vi "GCode Parser - SoftMotion Example.vi"() -> ()   [LabVIEW 2017]
uses:
  Typedefs/Motion Parameters.ctl
  <vilib>/Motion/Express/_s/nimc.fb.straightLineMove.blendMode.ctl
  GCode Parser/GCode Command Cluster.ctl
  <vilib>/Math Plots/3D Math Plots/3D Scatter/3D Scatter XCtrl/3D Scatter.xctl
  <vilib>/Motion/Express/_s/nimc.ex.clearFaults.clearFaults.axis.vi
  <vilib>/Motion/Express/_s/nimc.ex.power.power.axis.vi
  <vilib>/Motion/Express/_s/nimc.ex.resetPosition.resetPosition.axis.vi
  <vilib>/Motion/Express/_s/nimc.ex.straightLineMove.startStraightLineMove.coordinate.modeAbsolute.blendEnable.1.vi
  <vilib>/Motion/Express/_s/nimc.ex.arcMove.startArcMove.coordinate.modeCircular.blendEnable.1.vi
  <vilib>/Motion/Express/_s/nimc.ex.stopMove.stop.coordinate.modeDecelerate.vi
  <vilib>/Motion/Express/_s/nimc.ex.read.readTrajectoryData.coordinate.vi
  <vilib>/Motion/Express/_s/nimc.ex.read.readExecutionData.axis.vi
  <vilib>/Math Plots/3D Math Plots/3D Scatter/3D Scatter Datatype/Public/Plot Helper (Vector).vi
  <vilib>/Motion/BlockNode/FB.NIMotion.xnode
  <vilib>/Motion/Express/_s/nimc.fb.arcMove.blendMode.ctl
  <vilib>/Math Plots/3D Math Plots/3D Scatter/3D Scatter Datatype/3D Scatter Datatype.lvclass
panel:
  out "Array 2":string[](array[string])
  out "3D Scatter":refnum<class "3D Plot Datatype.lvclass">[](xcontrol)
  out "Array":dbl[](array[numeric])
  out "Current GCode Command":T1
  in  "Motion Parameters":T2={"timeout"=-1.0, "acceleration"=10000.0, "deceleration"=10000.0, "accel. jerk"=100000.0, "decel. jerk"=100000.0, "blend mode"=10551334, "blend delay"=-1.0, "smoothing"=0.5, "last blend"=FALSE} {"blend mode" items=["At Profile Complete"=10551335, "At Deceleration"=10551334, "After Delay"=10551336]}
  in  "G0 Velocity":dbl=20.0
  in  "Position Scale":dbl=1.0
  in  "Velocity Scale":dbl=1.0
  out "Global Stop":bool
  out "text":string
  in  "Quit":bool
  out "Iterations":i32
  out "Command Array":T1[](array[typedef])
  out "error out":errorcluster
  in  "start index":i32
  # "Be sure select \nafter delay"
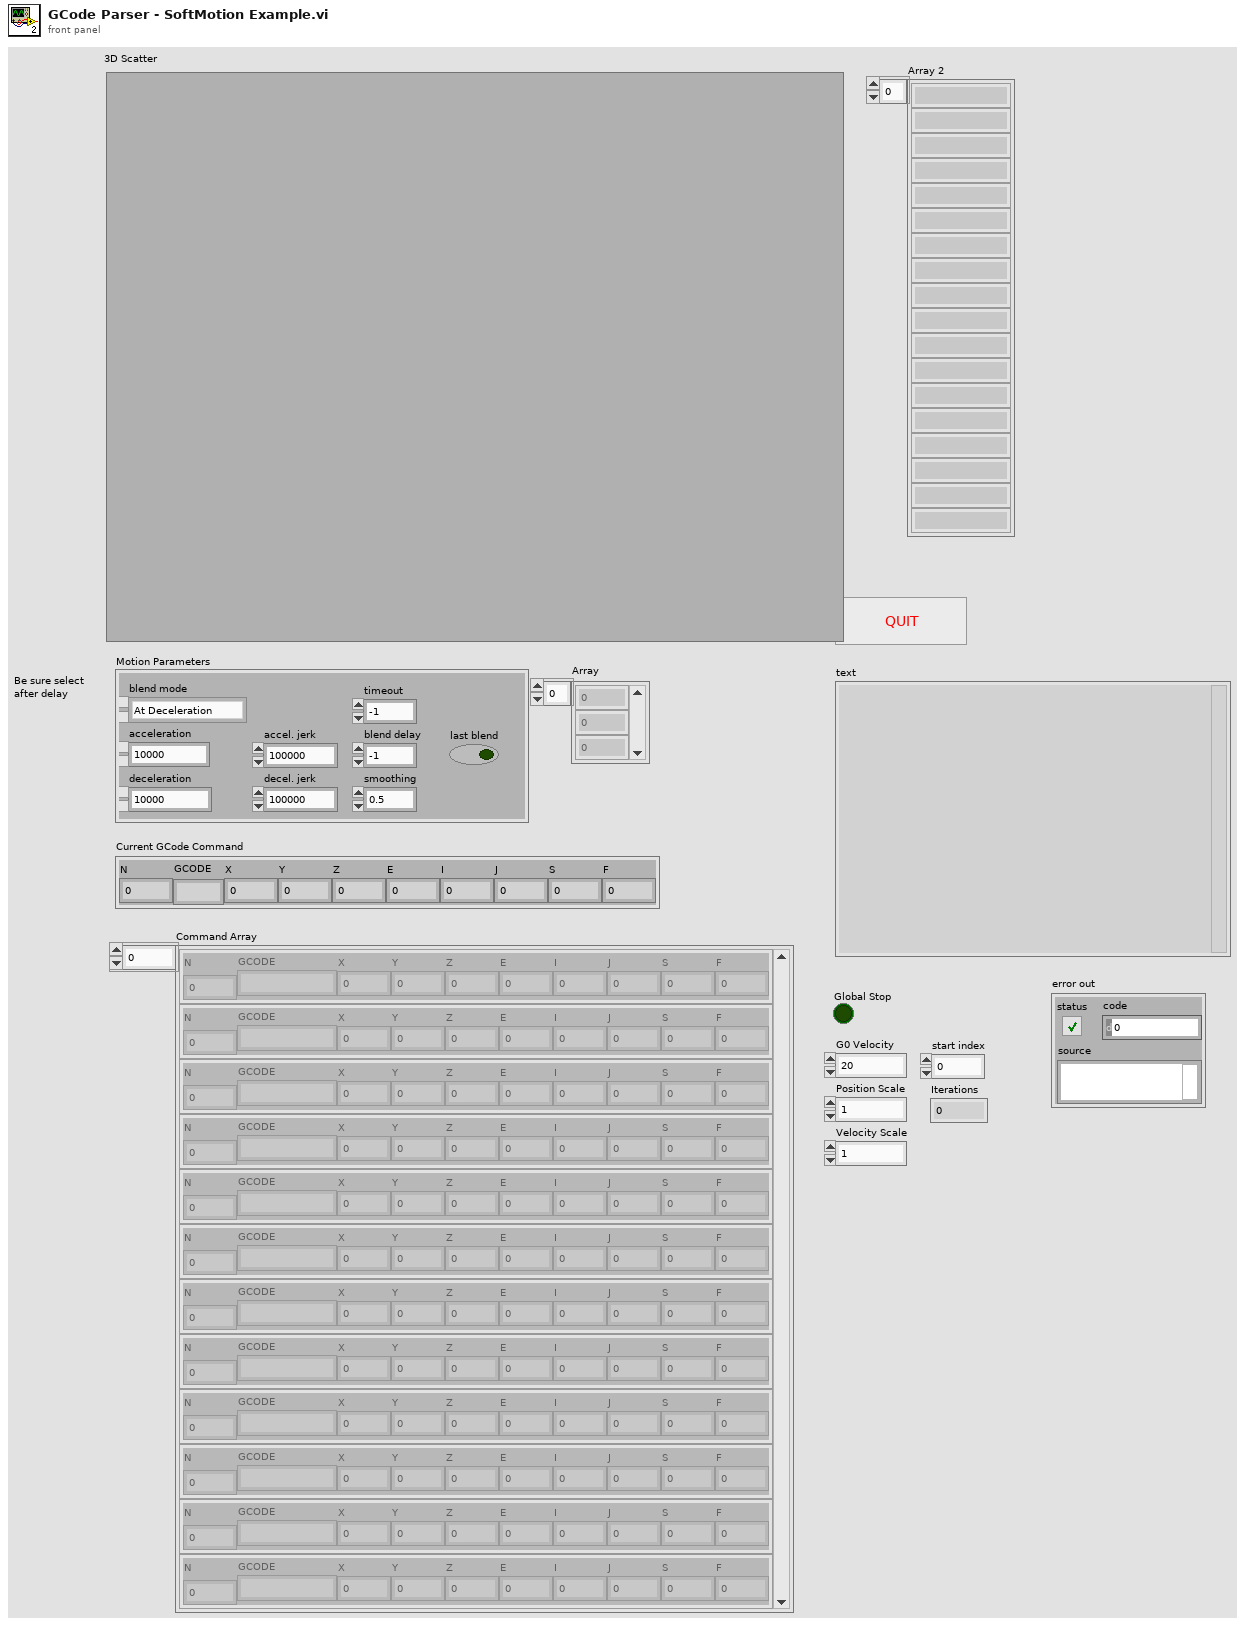
[diagram p1: front panel]
types:
  T1 = typedef "GCode Command Cluster.ctl" = cluster{"N":dbl, "GCODE":string, "X":dbl, "Y":dbl, "Z":dbl, "E":dbl, "I":dbl, "J":dbl, "S":dbl, "F":dbl}
  T2 = typedef "Motion Parameters.ctl" = cluster{"timeout":dbl, "acceleration":dbl, "deceleration":dbl, "accel. jerk":dbl, "decel. jerk":dbl, "blend mode":T3, "blend delay":dbl, "smoothing":dbl, "last blend":bool}
  T3 = typedef "nimc.fb.straightLineMove.blendMode.ctl" = i32
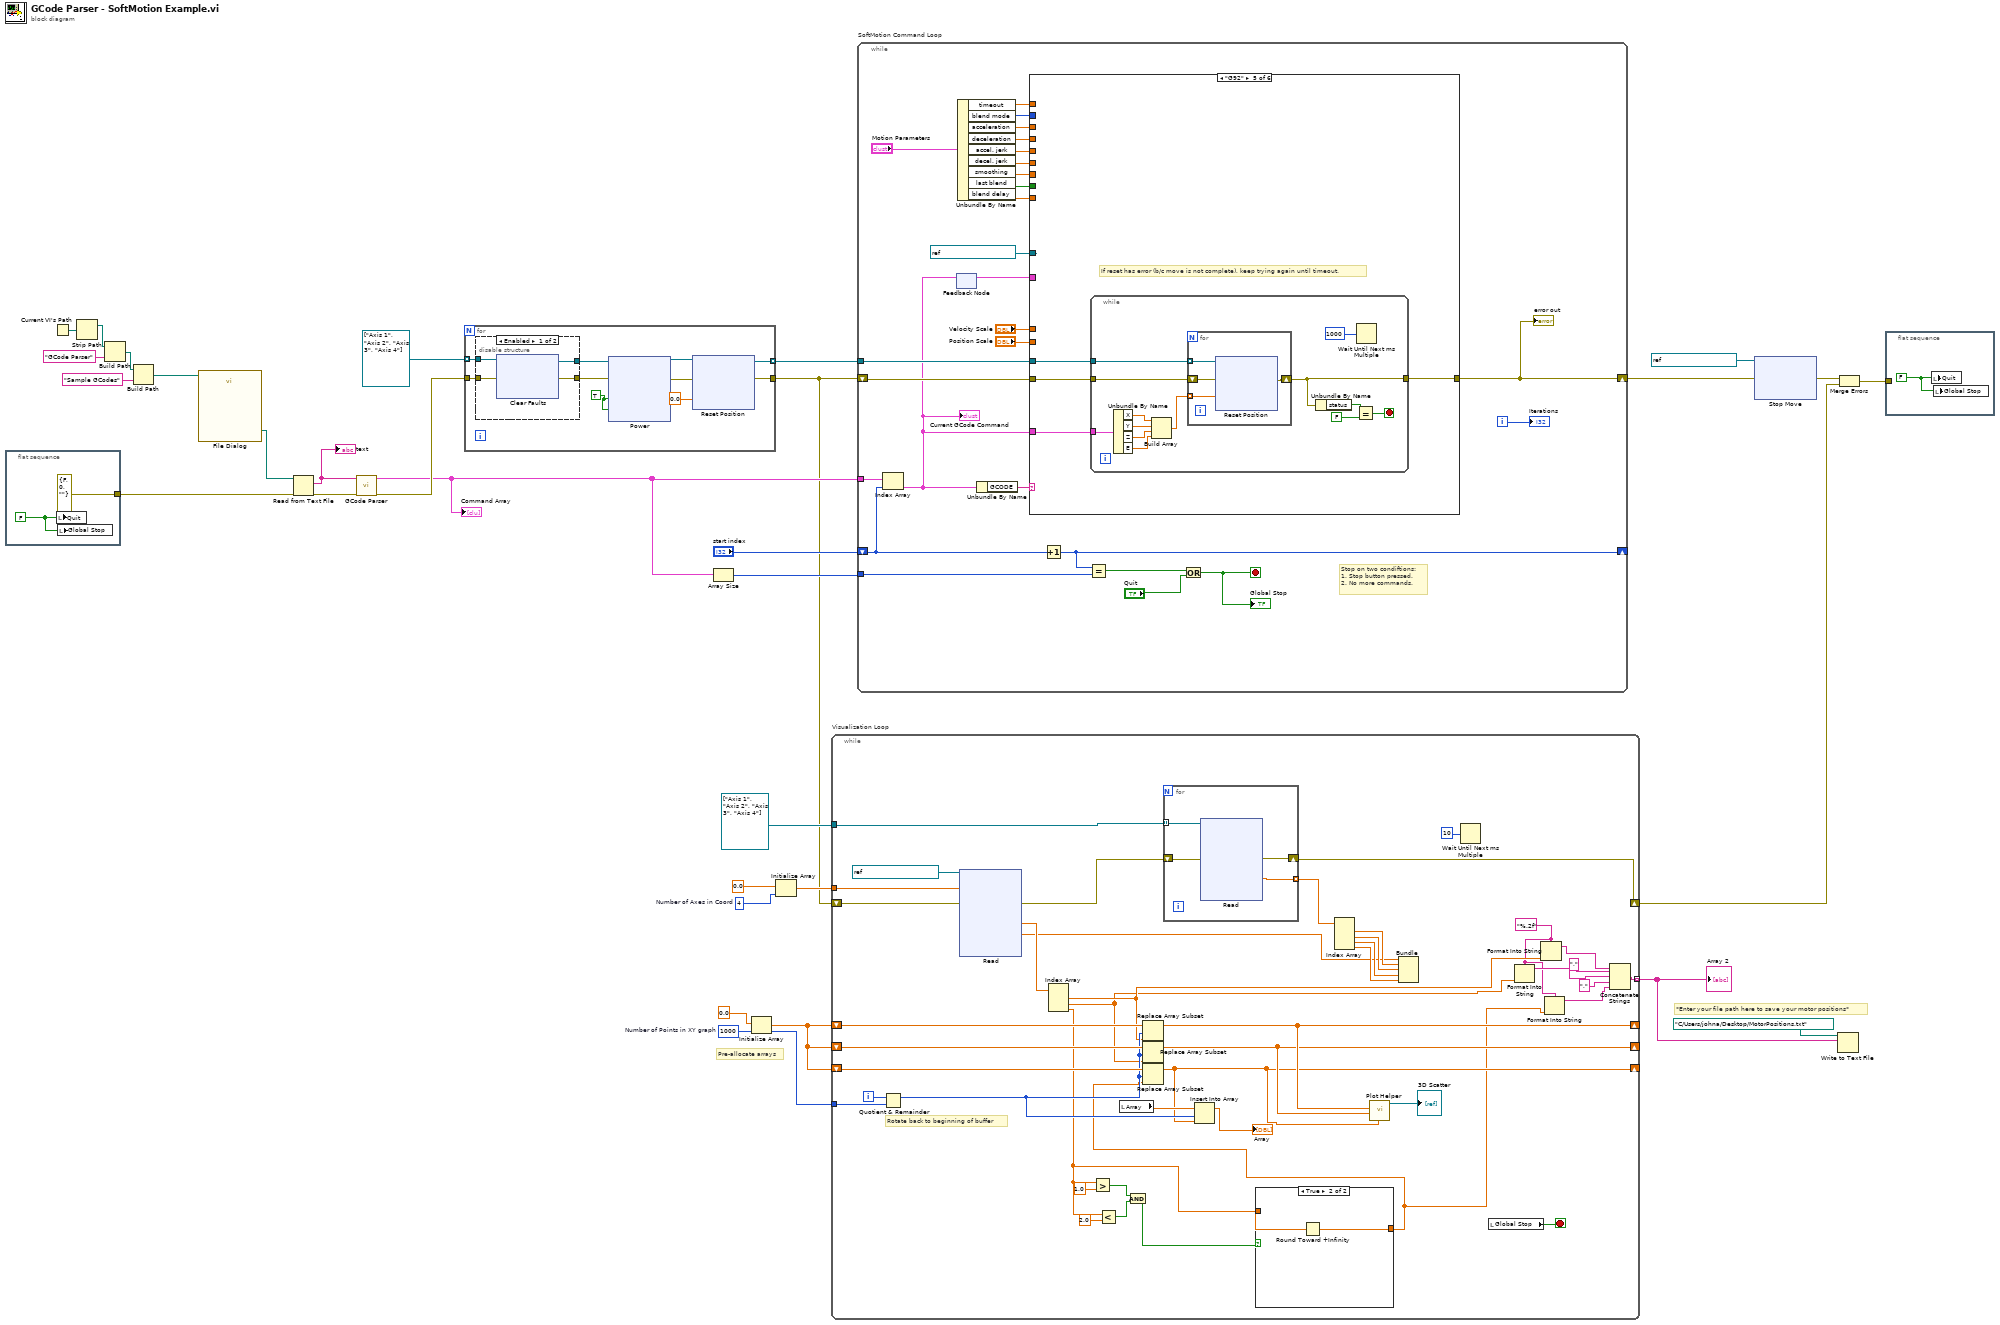
[diagram p0: block diagram]
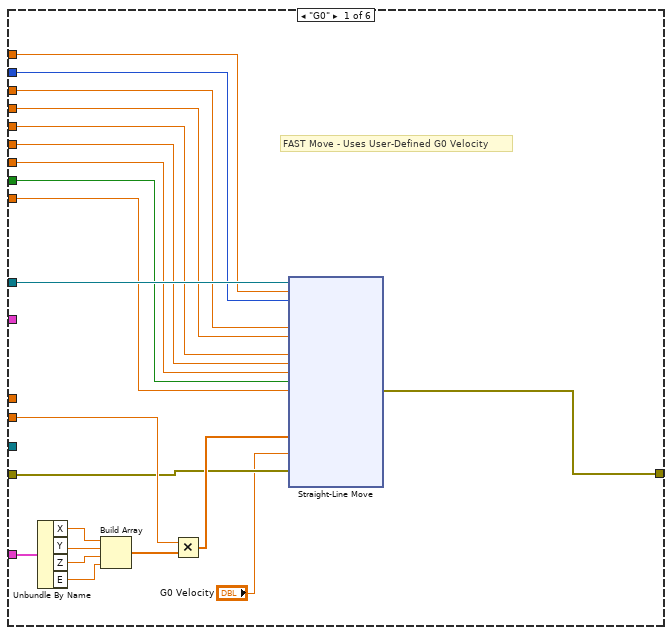
[diagram p2: hidden frame]
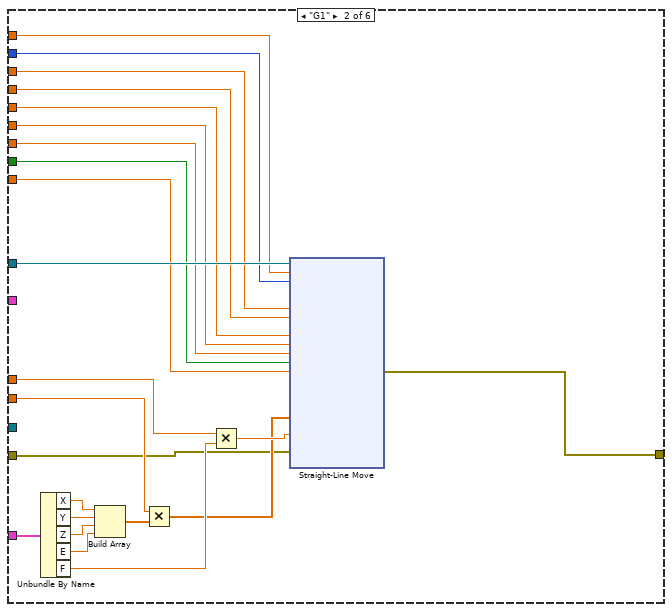
[diagram p3: hidden frame]
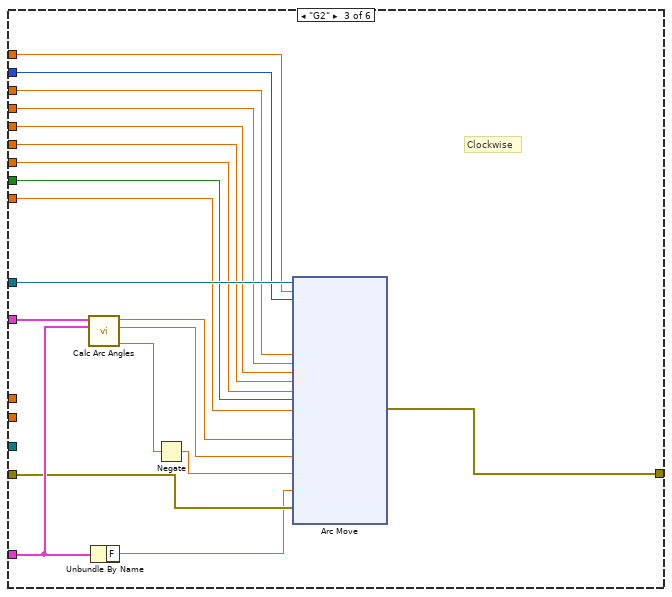
[diagram p4: hidden frame]
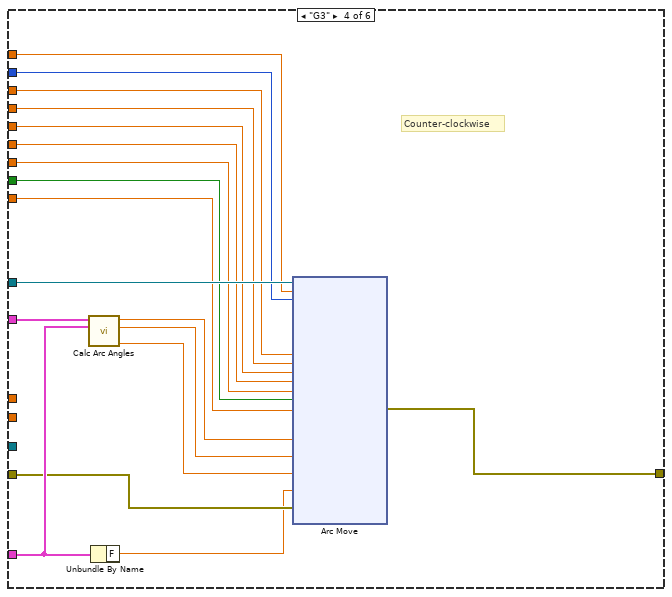
[diagram p5: hidden frame]
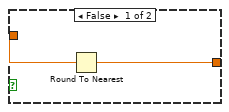
[diagram p7: hidden frame]
diagram:
  w27 = 1000  # Number of Points in XY graph
  w29 = 4  # Number of Axes in Coord
  # "*Enter your file path here to save your motor positions*"
  # "Pre-allocate arrays"
  n1 = flat-sequence {
    tunnel: [errorcluster {"status"=FALSE, "code"=0, "source"=""} ("error out")] -> w22
    frame #0 {
      w32 = FALSE ("Example Done")
      n2 = local write "Quit"(w32) -> ()
      n3 = local write "Global Stop"(w32) -> ()
    }
  }
  n4 = Current VI's Path() -> (path=w9:path)
  n5 = Strip Path(path=w9) -> (stripped path=w8:path)  [unwired: 1 out]
  n6 = Build Path(base path=w8, name or relative path="GCode Parser") -> (appended path=w4:path)
  n7 = Build Path(base path=w4, name or relative path="Sample GCodes") -> (appended path=w3:path)
  n8 = call "File Dialog"("start path"=w3) -> ("selected path"=w6:path)  [unwired: 11 in, 3 out]
  n9 = Read from Text File(file (use dialog)=w6, error in=w22) -> (text=w24:string, error out=w23:errorcluster)  [unwired: 2 in, 2 out]
  "text" <- w24
  n10 = call "GCode Parser.vi"("error in (no error)"=w23, "String in"=w24) -> ("error out"=w21:errorcluster, "Command Array"=w17:T1[])  [unwired: 8 in]
  "Command Array" <- w17
  n11 = for {
    tunnel: refnum<k21>[] ["Axis 1", "Axis 2", "Axis 3", "Axis 4"] -> [w43] mode=indexing
    tunnel: w21 -> [w42]
    tunnel: [w41] -> w14
    tunnel: [w34] -> w18 mode=indexing
    w36 = TRUE ("enable axis")
    n12 = disable-structure shown="Enabled" {
      disable-tunnel: w43 -> [w47 w53]
      disable-tunnel: w42 -> [w46 w52]
      disable-tunnel: [w45 w53] -> w39
      disable-tunnel: [w44 w52] -> w37
      frame Enabled {
        n13 = xnode ("Clear Faults")("resource"=w47, "error in"=w46) -> ("resource out"=w45:refnum<k21>, "error out"=w44:errorcluster)
      }
      frame Disabled {
      }
    }
    n14 = xnode ("Power")("enable axis"=w36, "enable drive"=w36, "resource"=w39, "error in"=w37) -> ("resource out"=w38:refnum<k21>, "error out"=w35:errorcluster)
    n15 = xnode ("Reset Position")("position"=0.0, "resource"=w38, "error in"=w35) -> ("resource out"=w34:refnum<k21>, "error out"=w41:errorcluster)
  }
  n16 = Array Size(array=w17) -> (size(s)=w16:i32)
  n17 = Initialize Array(0.0 ("element"), w27) -> (w26:dbl[])
  n18 = Initialize Array(0.0 ("element"), w29) -> (w25:dbl[])
  n19 = while "Visualization Loop" {
    shift-right: [w82] -> _
    shift-left: w26 -> [w110]
    shift-right: [w94] -> w13
    shift-left: w14 -> [w102]
    shift-right: [w81] -> _
    shift-left: w26 -> [w109]
    tunnel: w27 -> [w108]
    shift-right: [w80] -> _
    shift-left: w26 -> [w93]
    tunnel: w25 -> [w99]
    tunnel: refnum<k21>[] ["Axis 1", "Axis 2", "Axis 3", "Axis 4"] -> [w107]
    tunnel: [w76] -> w2 mode=indexing
    i -> [w91]
    stop <- w96 stop-if-true
    w69 = "%.2f" ("format string")
    # "Rotate back to beginning of buffer"
    n20 = Quotient & Remainder(x=w91, y=w108) -> (x-y*floor(x/y)=w89:i32)  [unwired: 1 out]
    n21 = xnode ("Read")("resource"=refnum<k21> "Coordinate Space 1" ("Motion Resource"), "commanded pos.[]"=w99, "error in"=w102) -> ("commanded pos.[] out"=w100:dbl[], "commanded vel."=w97:dbl, "error out"=w101:errorcluster)  [unwired: 3 out]
    n22 = Index Array(array=w100) -> (element #1=w75:dbl, element #2=w73:dbl, element #3=w79:dbl)  [unwired: 3 in]
    n23 = Greater?(x=w79, y=1.0) -> (0:w86:bool)
    n24 = Less?(x=w79, y=2.0) -> (x < y?=w85:bool)
    n25 = local read "Array"() -> (w90:dbl[])
    n26 = And(x=w86, y=w85) -> (x .and. y?=w84:bool)
    n27 = Replace Array Subset(array=w110, new element=w75, index=w89) -> (w82:dbl[])
    n28 = Replace Array Subset(array=w109, new element=w73, index=w89) -> (w81:dbl[])
    n29 = for {
      tunnel: w107 -> [w128] mode=indexing
      tunnel: [w127] -> w106 mode=indexing
      shift-right: [w125] -> w94
      shift-left: w101 -> [w126]
      n30 = xnode ("Read")("resource"=w128, "error in"=w126) -> ("velocity"=w127:dbl, "error out"=w125:errorcluster)  [unwired: 5 out]
    }
    n31 = case shown="True" w84 {
      tunnel: w79 -> [w113 w115]
      tunnel: [w112 w114] -> w71
      frame False {
        n32 = Round To Nearest(number=w113) -> (nearest integer value=w112:dbl)
      }
      frame True {
        n33 = Round Toward +Infinity(x=w115) -> (ceil(x): smallest int >= x=w114:dbl)
      }
    }
    n34 = Replace Array Subset(array=w93, new element=w71, index=w89) -> (w80:dbl[])
    n35 = Insert Into Array(array=w90, index=w89, new element=w80) -> (→"Array":dbl[])
    n36 = Index Array(array=w106) -> (element #1=w105:dbl, element #2=w104:dbl, element #3=w103:dbl, element #4=w98:dbl)  [unwired: 4 in]
    n37 = call-poly <vilib>:"Plot Helper.vi"("z vector"=w80, "y vector"=w81, "x vector"=w82) -> ("3D Plot lvclass Array out"=→"3D Scatter":refnum<class "3D Plot Datatype.lvclass">[])  [unwired: 3 in, 5 out]
    n38 = Bundle("commanded vel."=w97, "velocity"=w105, "velocity"=w104, "velocity"=w103, "velocity"=w98) -> ()  [unwired: 1 in, 1 out]
    n39 = Wait Until Next ms Multiple(millisecond multiple=u32 10) -> ()  [unwired: 1 out]
    n40 = local read "Global Stop"() -> (w96:bool)
    n41 = Format Into String(format string=w69, w73) -> (resulting string=w72:string)  [unwired: 2 in, 1 out]
    n42 = Format Into String(format string=w69, w75) -> (resulting string=w74:string)  [unwired: 2 in, 1 out]
    n43 = Format Into String(format string=w69, w71) -> (resulting string=w70:string)  [unwired: 2 in, 1 out]
    n44 = Concatenate Strings(w74, "," ("element"), w72, "," ("element"), w70) -> (w76:string)
  }
  "Array 2" <- w2
  n45 = while "SoftMotion Command Loop" {
    tunnel: w17 -> [w157]
    shift-right: [w154] -> _
    shift-left: "start index" -> [w156]
    shift-right: [w161] -> w11
    shift-left: w14 -> [w160]
    tunnel: w18 -> [w159]
    tunnel: w16 -> [w155]
    i -> [w158]
    stop <- w152 stop-if-true
    # "Stop on two condiftions:\n1. Stop button pressed.\n2. No more commands."
    n46 = Index Array(array=w157, index=w156) -> (element=w138:T1)
    "Current GCode Command" <- w138
    n47 = feedback-in #1(w138) -> ()
    n48 = feedback #1() -> (w139:T1)  [unwired: 1 in]
    n49 = Unbundle By Name("Motion Parameters") -> ("timeout"=w148:dbl, "blend mode"=w147:T3, "acceleration"=w146:dbl, "deceleration"=w145:dbl, "accel. jerk"=w144:dbl, "decel. jerk"=w143:dbl, "smoothing"=w141:dbl, "last blend"=w142:bool, "blend delay"=w140:dbl)
    n50 = Unbundle By Name(w138) -> ("GCODE"=w164:string)
    n51 = case shown="\"G92\"" w164 {
      tunnel: refnum<k21> "Coordinate Space 1" ("Motion Resource") -> [w177 w219 w267 w307 _ _]
      tunnel: [w185 w228 w257 w297 w330 w356] -> w161
      tunnel: "Velocity Scale" -> [_ w207 _ _ _ _]
      tunnel: w138 -> [w180 w223 w264 w304 w331 _]
      tunnel: "Position Scale" -> [w178 w220 _ _ _ _]
      tunnel: w160 -> [w175 w217 w258 w298 w332 w356]
      tunnel: w148 -> [w174 w216 w263 w303 _ _]
      tunnel: w147 -> [w173 w215 w249 w291 _ _]
      tunnel: w146 -> [w172 w214 w262 w302 _ _]
      tunnel: w145 -> [w171 w213 w261 w301 _ _]
      tunnel: w144 -> [w170 w212 w260 w300 _ _]
      tunnel: w143 -> [w169 w211 w259 w299 _ _]
      tunnel: w141 -> [w168 w210 w250 w292 _ _]
      tunnel: w142 -> [w167 w209 w251 w293 _ _]
      tunnel: w140 -> [w166 w208 w252 w294 _ _]
      tunnel: w159 -> [_ _ _ _ w333 _]
      tunnel: w139 -> [_ _ w266 w306 _ _]
      frame "G0" {
        # "FAST Move - Uses User-Defined G0 Velocity"
        n52 = Unbundle By Name(w180) -> ("X"=w184:dbl, "Y"=w183:dbl, "Z"=w182:dbl, "E"=w181:dbl)
        n53 = Build Array(w184, w183, w182, w181) -> (w179:dbl[])
        n54 = Multiply(x=w178, y=w179) -> (x*y=w176:dbl[])
        n55 = xnode ("Straight-Line Move")("position[]"=w176, "velocity"="G0 Velocity", "error in"=w175, "resource"=w177, "timeout"=w174, "blend mode"=w173, "acceleration"=w172, "deceleration"=w171, "accel. jerk"=w170, "decel. jerk"=w169, "smoothing"=w168, "last blend"=w167, "blend delay"=w166) -> ("error out"=w185:errorcluster)  [unwired: 2 out]
      }
      frame "G1" {
        n56 = Unbundle By Name(w223) -> ("X"=w227:dbl, "Y"=w226:dbl, "Z"=w206:dbl, "E"=w225:dbl, "F"=w224:dbl)
        n57 = Build Array(w227, w226, w206, w225) -> (w221:dbl[])
        n58 = Multiply(x=w220, y=w221) -> (x*y=w218:dbl[])
        n59 = Multiply(x=w207, y=w224) -> (x*y=w222:dbl)
        n60 = xnode ("Straight-Line Move")("position[]"=w218, "velocity"=w222, "error in"=w217, "resource"=w219, "timeout"=w216, "blend mode"=w215, "acceleration"=w214, "deceleration"=w213, "accel. jerk"=w212, "decel. jerk"=w211, "smoothing"=w210, "last blend"=w209, "blend delay"=w208) -> ("error out"=w228:errorcluster)  [unwired: 2 out]
      }
      frame "G2" {
        # "Clockwise"
        n61 = call "Calc Arc Angles.vi"("Arc CMD"=w264, "Initial CMD"=w266) -> ("travel angle out"=w255:dbl, "start angle (tangent)"=w254:dbl, "R"=w265:dbl)  [unwired: 7 in]
        n62 = Unbundle By Name(w264) -> ("F"=w253:dbl)
        n63 = Negate(x=w255) -> (-x=w256:dbl)
        n64 = xnode ("Arc Move")("radius"=w265, "start angle"=w254, "travel angle"=w256, "velocity"=w253, "error in"=w258, "resource"=w267, "timeout"=w263, "blend mode"=w249, "acceleration"=w262, "deceleration"=w261, "accel. jerk"=w260, "decel. jerk"=w259, "smoothing"=w250, "last blend"=w251, "blend delay"=w252) -> ("error out"=w257:errorcluster)  [unwired: 2 out]
      }
      frame "G3" {
        # "Counter-clockwise"
        n65 = call "Calc Arc Angles.vi"("Arc CMD"=w304, "Initial CMD"=w306) -> ("travel angle out"=w290:dbl, "start angle (tangent)"=w296:dbl, "R"=w305:dbl)  [unwired: 7 in]
        n66 = Unbundle By Name(w304) -> ("F"=w295:dbl)
        n67 = xnode ("Arc Move")("radius"=w305, "start angle"=w296, "travel angle"=w290, "velocity"=w295, "error in"=w298, "resource"=w307, "timeout"=w303, "blend mode"=w291, "acceleration"=w302, "deceleration"=w301, "accel. jerk"=w300, "decel. jerk"=w299, "smoothing"=w292, "last blend"=w293, "blend delay"=w294) -> ("error out"=w297:errorcluster)  [unwired: 2 out]
      }
      frame "G92" {
        # "If reset has error (b/c move is not complete), keep trying again until timeout."
        n68 = while {
          tunnel: [w343] -> w330
          tunnel: w333 -> [w341]
          tunnel: w332 -> [w340]
          tunnel: w331 -> [w335]
          stop <- w342 stop-if-true
          n69 = Unbundle By Name(w335) -> ("X"=w339:dbl, "Y"=w338:dbl, "Z"=w337:dbl, "E"=w336:dbl)
          n70 = Build Array(w339, w338, w337, w336) -> (w334:dbl[])
          n71 = for {
            tunnel: w341 -> [w349] mode=indexing
            shift-right: [w350] -> w343
            shift-left: w340 -> [w348]
            tunnel: w334 -> [w347] mode=indexing
            n72 = xnode ("Reset Position")("position"=w347, "resource"=w349, "error in"=w348) -> ("error out"=w350:errorcluster)  [unwired: 1 out]
          }
          n73 = Unbundle By Name(w343) -> ("status"=w345:bool)
          n74 = Equal?(x=w345, y=FALSE) -> (x = y?=w342:bool)
          n75 = Wait Until Next ms Multiple(millisecond multiple=u32 1000) -> ()  [unwired: 1 out]
        }
      }
      frame Default {
        # "Empty case for all other codes."
      }
    }
    "error out" <- w161
    n76 = Increment(x=w156) -> (x+1=w154:i32)
    n77 = Equal?(x=w154, y=w155) -> (x = y?=w153:bool)
    n78 = Or(x=w153, y="Quit") -> (x .or. y?=w152:bool)
    "Global Stop" <- w152
    "Iterations" <- w158
  }
  n79 = xnode ("Stop Move")("resource"=refnum<k21> "Coordinate Space 1" ("coordinate"), "error in"=w11) -> ("error out"=w10:errorcluster)  [unwired: 1 in, 2 out]
  n80 = Write to Text File(file (use dialog)=path "C:/Users/johna/Desktop/MotorPositions.txt", text=w2) -> ()  [unwired: 2 in, 3 out]
  n81 = Merge Errors(w10, w13) -> (w15:errorcluster)
  n82 = flat-sequence {
    tunnel: w15 -> [_]
    frame #0 {
      w357 = FALSE ("Example Done")
      n83 = local write "Quit"(w357) -> ()
      n84 = local write "Global Stop"(w357) -> ()
    }
  }
